vi "Start Data Logger.vi"(11 "Application in":refnum<class "Application.lvclass">) -> (3 "Application out":refnum<class "Application.lvclass">)   [LabVIEW 2017, in "Application.lvlib" / "Application.lvclass"]
uses:
  Application.lvclass
  <vilib>/TSS/ACRObat Test Framework/Core Launcher/Core Manager Methods -- Enum.ctl
  <vilib>/TSS/ACRObat Test Framework/Classes/Data/Data Logger/Class/Data Logger.lvclass
  <vilib>/TSS/ACRObat Test Framework/Core Launcher/Core Launcher.lvlib
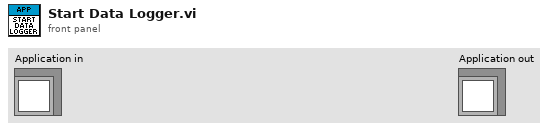
[diagram p1: front panel]
types:
  T1 = typedef "Core Launcher.lvlib/Core Manager Methods -- Enum.ctl" = enum16{"Spawn Objects", "Get Objects", "Destroy Objects"}
  T2 = typedef "Application.lvlib/App Settings.lvclass/Class Settings -- Cluster.ctl" = cluster{"DataLogging Enabled":bool, "AutoStart":bool, "AutoClear":bool, "Cycle Timeout":u32, "Wait Before Clear":u32, "Machine ID":string, "Test Type":string, "Product Name":string, "Meta Tags":string[], "Meta Values":string[], "Viewer Settings":cluster{"DataViewer Headers":string[], "Pass Fail Settings":T3}}
  T3 = typedef "Data Viewer.lvlib/Data Viewer Settings.lvclass/Pass Fail Criteria -- Cluster.ctl" = cluster{"Header":string, "Criteria":string}
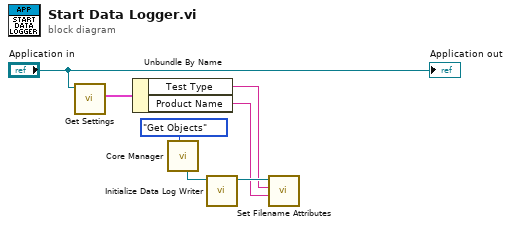
[diagram p0: block diagram]
diagram:
  n1 = call "Get Settings.vi"("Acrobat Template in"="Application in") -> ("Settings"=w3:T2)  [unwired: 8 in, 2 out]
  n2 = Unbundle By Name(w3) -> ("Test Type"=w2:string, "Product Name"=w1:string)
  n3 = call <vilib>:"Core Manager.vi"("Method"=Core_Manager_Methods_--_Enum."Get Objects") -> ("DataLogger"=w6:refnum<class "Data Logger.lvclass">)  [unwired: 6 in, 4 out]
  n4 = call-dynamic "Initialize Data Log Writer.vi"("DataLogger in"=w6) -> ("DataLogger out"=w7:refnum<class "Data Logger.lvclass">)  [unwired: 9 in, 1 out]
  n5 = call <vilib>:"Set Filename Attributes.vi"("Product Name"=w1, "Product Type"=w2, "DataLogger in"=w7) -> ()  [unwired: 7 in, 2 out]
  "Application out" <- "Application in"
